vi "Restart.vi"(8 "error in (no error)":errorcluster, 11 "MJPEG Reader in":refnum<data-value>) -> (0 "error out":errorcluster, 3 "MJPEG Reader out":refnum<data-value>)   [LabVIEW 2015, in "MJPEG Reader.lvclass"]
doc: "Restarts the MJPEG Reader."
uses:
  MJPEG Reader.lvclass
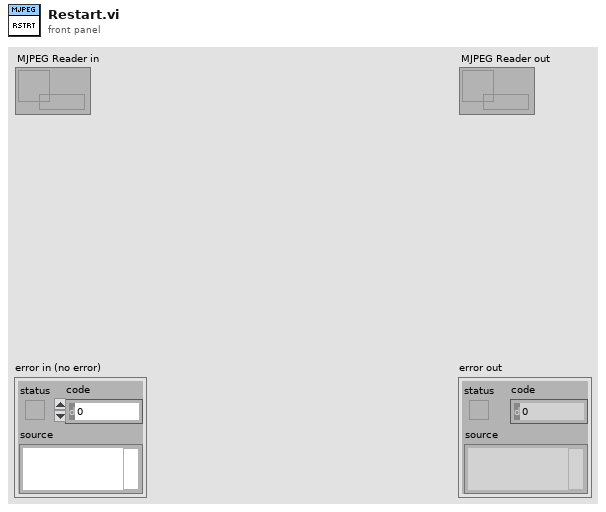
[diagram p1: front panel]
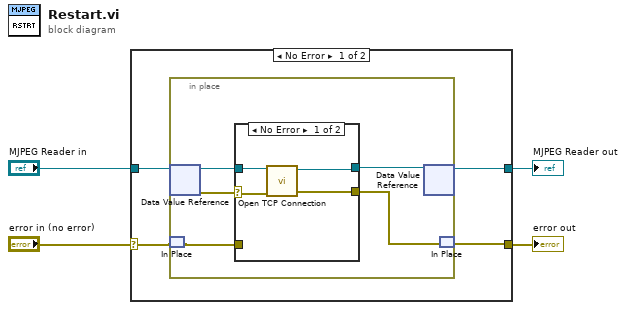
[diagram p0: block diagram]
diagram:
  n1 = case shown="No Error" "error in (no error)" {
    selector: "error in (no error)" -> [w7 w21]
    tunnel: [w6 w21] -> w3
    tunnel: [w5 w20] -> w1
    tunnel: "MJPEG Reader in" -> [w8 w20]
    frame No Error {
      n2 = in-place {
        n3 = in-place-dvr #1(w8) -> (w12:refnum<class "MJPEG Reader.lvclass">, w13:errorcluster)
        n4 = in-place-match #2(w7) -> (w10:errorcluster)
        n5 = case shown="No Error" w13 {
          selector: w13 -> [w16 w18]
          tunnel: w12 -> [w17 w19]
          tunnel: w10 -> [_ _]
          tunnel: [w15 w19] -> w11
          tunnel: [w14 w18] -> w9
          frame No Error {
            n6 = call "Open TCP Connection.vi"("error in (no error)"=w16, "MJPEG Reader in"=w17) -> ("error out"=w14:errorcluster, "MJPEG Reader out"=w15:refnum<class "MJPEG Reader.lvclass">)  [unwired: 8 in]
          }
          frame Error {
          }
        }
        n7 = in-place-dvr #1(w11) -> (w5:refnum<data-value>)  [unwired: 1 out]
        n8 = in-place-match #2(w9) -> (w6:errorcluster)
      }
    }
    frame Error {
    }
  }
  "error out" <- w3
  "MJPEG Reader out" <- w1
